vi "readSerial.vi"(2 "Serial Settings:Baud Rate":u32=921600, 3 "Termination Character":string caption="Termination Character (0D: Carriage Return)", 4 "VISA resource name":refnum<visa-resource-name>) -> (0 "Response String":string)   [LabVIEW 2014]
panel:
  in  "Allowed Byte Count":u32=100 caption="Max-Allowed Byte Count (100)"
  in  "Timeout":u32=1000 caption="Timeout Time, ms (1000)"
  in  "error in (no error)":errorcluster
  out "error out":errorcluster
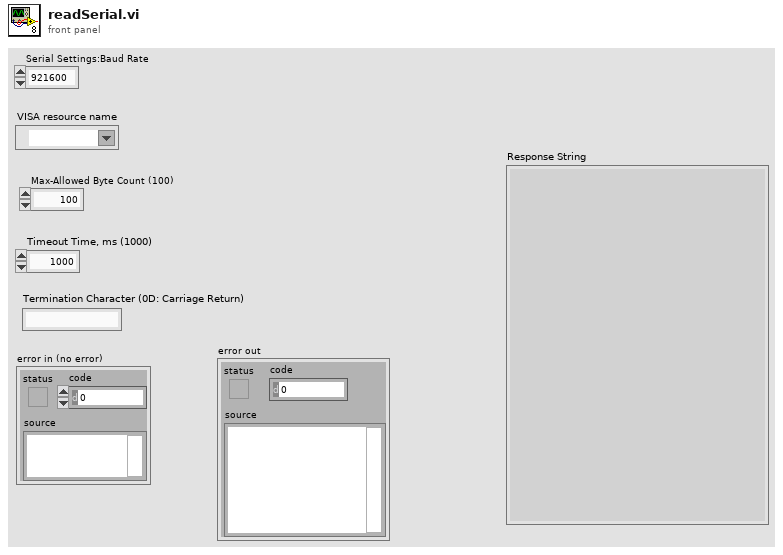
[diagram p1: front panel]
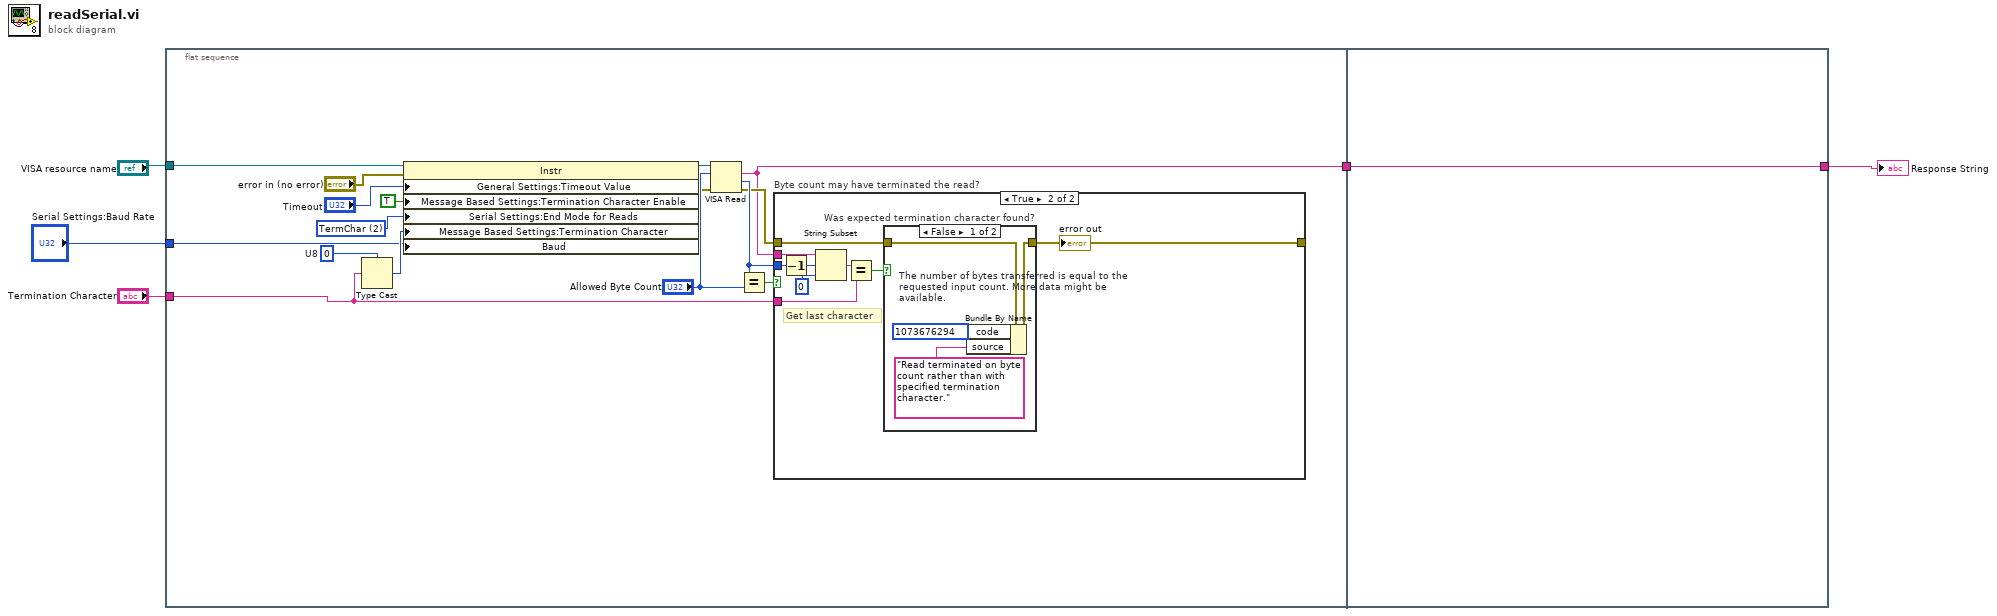
[diagram p0: block diagram]
diagram:
  n1 = flat-sequence {
    tunnel: "VISA resource name" -> [w10]
    tunnel: "Termination Character" -> [w9]
    tunnel: [w8] -> w2
    tunnel: "Serial Settings:Baud Rate" -> [w6]
    tunnel: [w38] -> w3
    tunnel: w2 -> [w38]
    frame #0 {
      w20 = u8 0  # U8
      w22 = u16 2 items=["None", "LastBit", "TermChar"] ("Serial Settings:Serial End Mode for Reads")
      n2 = Type Cast(type=w20, x=w9) -> (*(type *) &x=w19:u8)
      n3 = property class="Instr"(reference=w10, error in="error in (no error)", "General Settings:Timeout Value"="Timeout", "Message Based Settings:Termination Character Enable"=TRUE, "Serial Settings:End Mode for Reads"=w22, "Message Based Settings:Termination Character"=w19, "Baud"=w6) -> (reference out=w7:refnum<visa-resource-name>, error out=w13:errorcluster)
      n4 = VISA Read(VISA resource name=w7, byte count="Allowed Byte Count", error in (no error)=w13) -> (read buffer=w8:string, return count=w18:u32, error out=w17:errorcluster)  [unwired: 1 out]
      n5 = Equal?(x=w18, y="Allowed Byte Count") -> (x = y?=w21:bool)
      n6 = case "Byte count may have terminated the read?" shown="True" w21 {
        tunnel: w17 -> [w23 w32]
        tunnel: [w23 w31] -> w11
        tunnel: w8 -> [_ w30]
        tunnel: w18 -> [_ w29]
        tunnel: w9 -> [_ w25]
        frame False {
        }
        frame True {
          # "Get last character"
          n7 = Decrement(x=w29) -> (x-1=w24:u32)
          n8 = String Subset(string=w30, offset (0)=w24, length (rest)=0 ("length (rest)")) -> (substring=w27:string)
          n9 = Equal?(x=w27, y=w25) -> (x = y?=w26:bool)
          n10 = case "Was expected termination character found?" shown="False" w26 {
            tunnel: w32 -> [w36 w37]
            tunnel: [w35 w37] -> w31
            frame False {
              w34 = 1073676294  # The number of bytes transferred is equal to the requested input count. More data might be available.
              n11 = Bundle By Name(cluster=w36, "code"=w34, "source"="Read terminated on byte count rather than with specified termination character.") -> (w35:errorcluster)
            }
            frame True {
            }
          }
        }
      }
      "error out" <- w11
    }
    frame #1 {
    }
  }
  "Response String" <- w3
